vi "Run.vi"(8 "error in (no error)":errorcluster, 11 "LabBOT in":refnum<class "LabBOT.lvclass">) -> (0 "error out":errorcluster, 3 "LabBOT out":refnum<class "LabBOT.lvclass">)   [LabVIEW 2020, in "Rover.lvlib" / "LabBOT.lvclass"]
uses:
  LabBOT.lvclass
  nmea/nmea/nmea/Full Data.ctl
  nmea/nmea/nmea/Fix.ctl
  nmea/nmea/nmea/Velocity.ctl
  nmea/nmea/nmea/DOP.ctl
  nmea/nmea/nmea/Satellite.ctl
  nmea/nmea/nmea/Fix Type.ctl
  nmea/nmea/nmea/Fix Mode.ctl
  bno055/BNO055/BNO055/Euler Angles.ctl
  bno055/BNO055/BNO055/Calibration Status.ctl
  LabBOT.lvclass/LabBOT.ctl
  bno055/BNO055/BNO055/BNO055.lvclass
  nmea/nmea/nmea/nmea.lvclass
  nmea/nmea/VISA GPS/VISA GPS.lvclass
panel:
  in  "stop":bool
  out "Calibration Status":T1
  out "Euler Angles":T2
  out "Full Data":T3 {"Fix"."Longitude" format="%_16f"; "Fix"."Latitude" format="%_16f"}
  # "CENSORED"
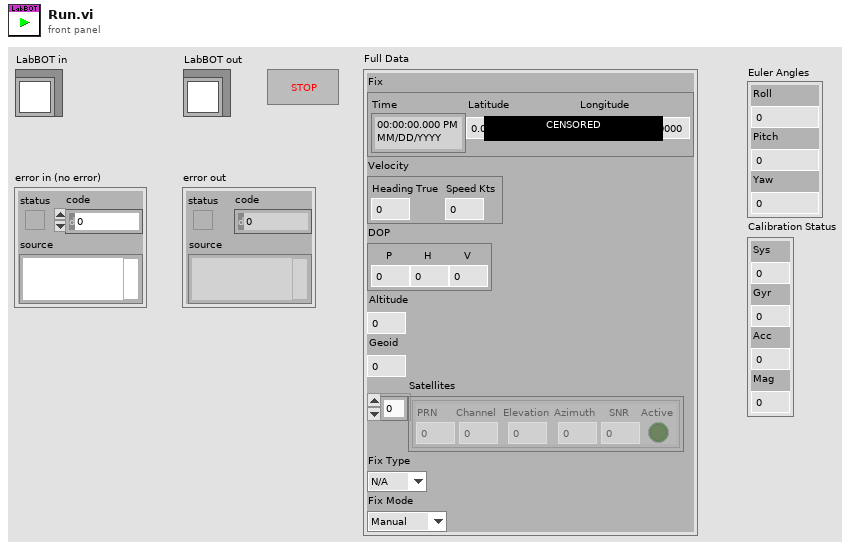
[diagram p1: front panel]
types:
  T1 = typedef "BNO055.lvlib/BNO055.lvclass/Calibration Status.ctl" = cluster{"Sys":u8, "Gyr":u8, "Acc":u8, "Mag":u8}
  T2 = typedef "BNO055.lvlib/BNO055.lvclass/Euler Angles.ctl" = cluster{"Roll":dbl, "Pitch":dbl, "Yaw":dbl}
  T3 = typedef "nmea.lvlib/nmea.lvclass/Full Data.ctl" = cluster{"Fix":T4, "Velocity":T5, "DOP":T6, "Altitude":dbl, "Geoid":dbl, "Satellites":T7[], "Fix Type":T8, "Fix Mode":T9}
  T4 = typedef "nmea.lvlib/nmea.lvclass/Fix.ctl" = cluster{"Time":timestamp, "Latitude":dbl, "Longitude":dbl}
  T5 = typedef "nmea.lvlib/nmea.lvclass/Velocity.ctl" = cluster{"Heading True":dbl, "Speed Kts":dbl}
  T6 = typedef "nmea.lvlib/nmea.lvclass/DOP.ctl" = cluster{"P":dbl, "H":dbl, "V":dbl}
  T7 = typedef "nmea.lvlib/nmea.lvclass/Satellite.ctl" = cluster{"PRN":u8, "Channel":u8, "Elevation":u8, "Azimuth":u16, "SNR":u8, "Active":bool}
  T8 = typedef "nmea.lvlib/nmea.lvclass/Fix Type.ctl" = enum16{"N/A", "None", "2D", "3D"}
  T9 = typedef "nmea.lvlib/nmea.lvclass/Fix Mode.ctl" = enum16{"Manual", "Auto 2/3D"}
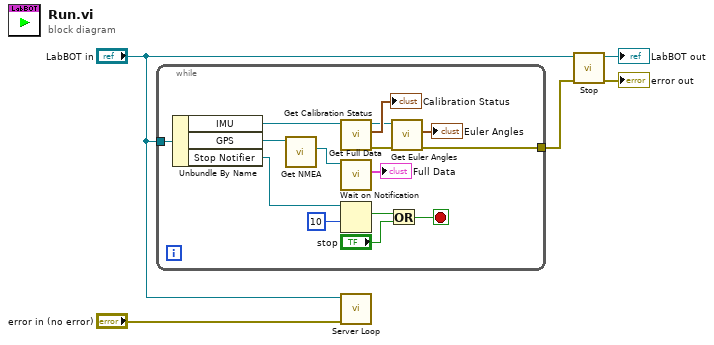
[diagram p0: block diagram]
diagram:
  n1 = while {
    tunnel: "LabBOT in" -> [w20]
    tunnel: [w11] -> w1
    stop <- w6 stop-if-true
    n2 = Unbundle By Name(w20) -> ("IMU"=w19:refnum<class "BNO055.lvclass">, "GPS"=w15:refnum<class "VISA GPS.lvclass">, "Stop Notifier"=w9:refnum<notifier>)
    n3 = call "Get NMEA.vi"("VISA GPS in"=w15) -> ("NMEA"=w14:refnum<class "nmea.lvclass">)  [unwired: 8 in, 2 out]
    n4 = call "Get Calibration Status.vi"("BNO055 in"=w19) -> ("error out"=w12:errorcluster, "Calibration Status"=→"Calibration Status":T1, "BNO055 out"=w17:refnum<class "BNO055.lvclass">)  [unwired: 8 in]
    n5 = call "Get Full Data.vi"("nmea in"=w14) -> ("Full Data"=→"Full Data":T3)  [unwired: 8 in, 2 out]
    n6 = Wait on Notification(notifier=w9, timeout in ms (-1)=10) -> (notification=w8:bool)  [unwired: 2 in, 3 out]
    n7 = Or(x=w8, y="stop") -> (x .or. y?=w6:bool)
    n8 = call "Get Euler Angles.vi"("error in (no error)"=w12, "BNO055 in"=w17) -> ("error out"=w11:errorcluster, "Euler Angles"=→"Euler Angles":T2)  [unwired: 7 in, 1 out]
  }
  n9 = call "Server Loop.vi"("error in (no error)"="error in (no error)", "LabBOT in"="LabBOT in") -> ()  [unwired: 9 in, 1 out]
  n10 = call "Stop.vi"("error in (no error)"=w1, "LabBOT in"="LabBOT in") -> ("error out"=→"error out":errorcluster, "LabBOT out"=→"LabBOT out":refnum<class "LabBOT.lvclass">)  [unwired: 8 in]
